vi "Broadcast Message Data.vi"(8 "error in (no error)":errorcluster, 10 "Message ID":u32, 11 "Debugger in":refnum<class "Debugger.lvclass">) -> (0 "error out":errorcluster, 3 "Debugger out":refnum<class "Debugger.lvclass">)   [LabVIEW 2020, in "Debugger.lvclass"]
uses:
  Debugger.lvclass
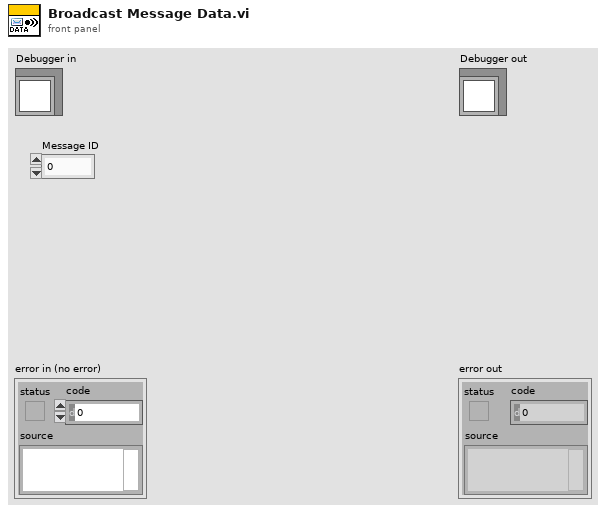
[diagram p1: front panel]
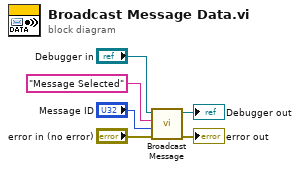
[diagram p0: block diagram]
diagram:
  n1 = call-dynamic "Broadcast Message.vi"("error in (no error)"="error in (no error)", "Message Data"="Message ID", "Message"="Message Selected", "Process In"="Debugger in") -> ("error out"=→"error out":errorcluster, "Process Out"=→"Debugger out":refnum<class "Debugger.lvclass">)  [unwired: 6 in]
